vi "Nominal-Gate TimeOF.vi"(7 "Item ID":string) -> (1 "Error":bool, 2 "Gate Time":string, 3 "Nominal Frequency":string)   [LabVIEW 2023]
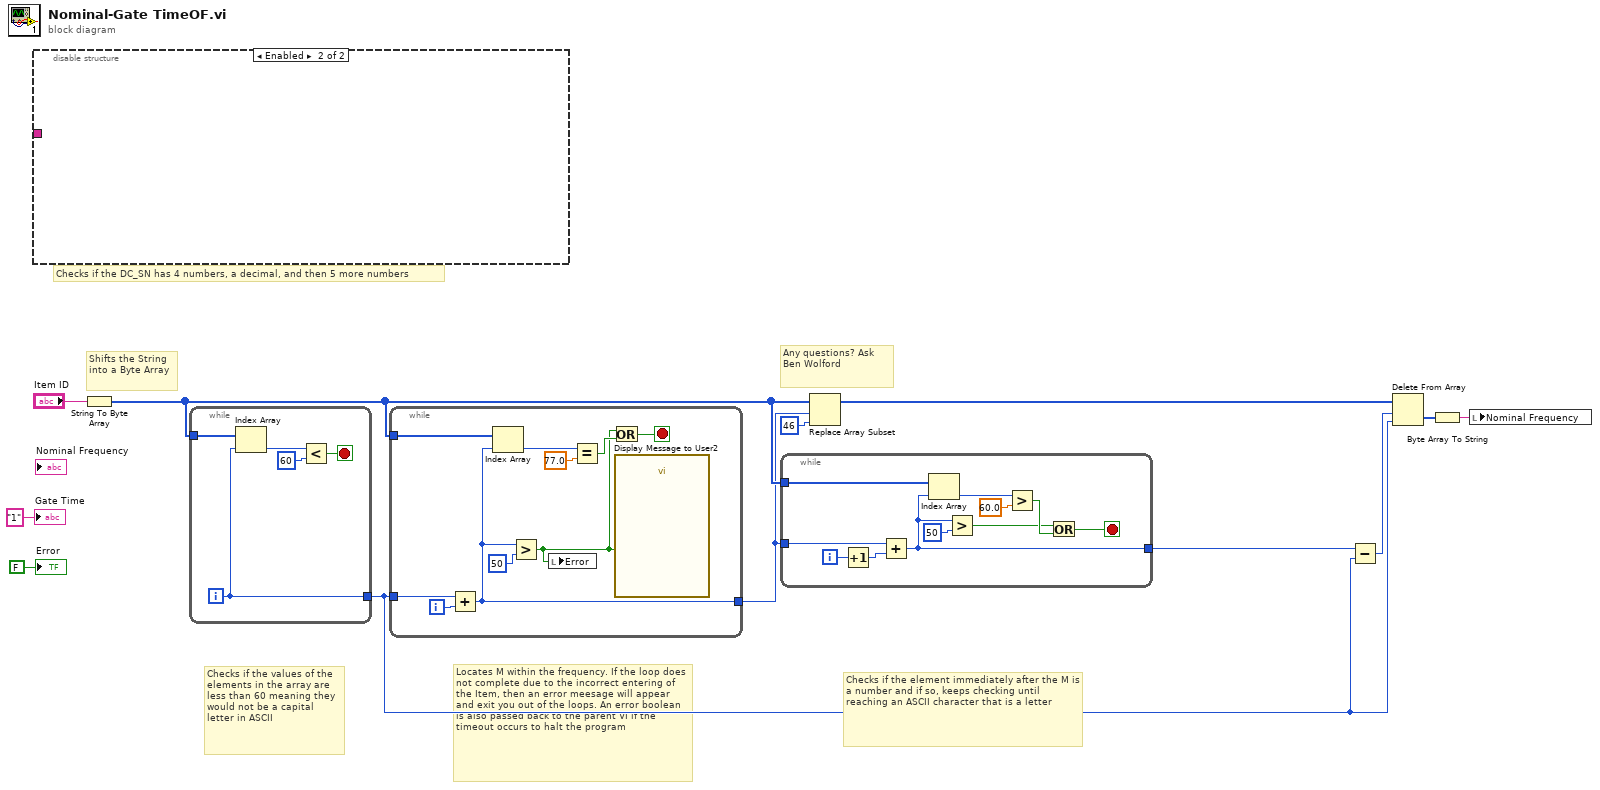
[diagram p0: block diagram]
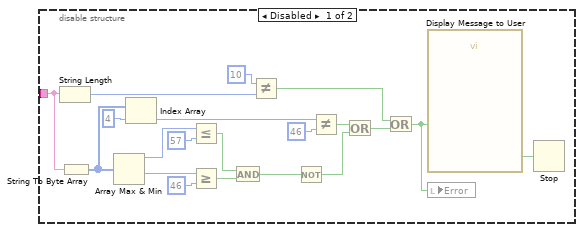
[diagram p2: hidden frame]
diagram:
  # "Checks if the element immediately after the M is a number and if so, keeps checking until reaching an ASCII character that is a letter"
  # "Locates M within the frequency. If the loop does not complete due to the incorrect entering of the Item, then an error meesage will appear and exit you out of the loops. An error boolean is also passed back to the parent VI if the timeout occurs to halt the program"
  # "Any questions? Ask Ben Wolford"
  # "Checks if the DC_SN has 4 numbers, a decimal, and then 5 more numbers"
  # "Checks if the values of the elements in the array are less than 60 meaning they would not be a capital letter in ASCII"
  # "Shifts the String into a Byte Array"
  n1 = disable-structure shown="Enabled" {
    disable-tunnel: _ -> [w13 _]
    frame Disabled {
      n2 = String Length(string=w13) -> (length=w19:i32)
      n3 = String To Byte Array(string=w13) -> (unsigned byte array=w26:u8[])
      n4 = Array Max & Min(array=w26) -> (max value=w28:u8, min value=w27:u8)  [unwired: 2 out]
      n5 = Index Array(array=w26, index=4) -> (element=w23:u8)
      n6 = Less Or Equal?(x=w28, y=u8 57) -> (x <= y?=w29:bool)
      n7 = Greater Or Equal?(x=w27, y=u8 46) -> (x >= y?=w30:bool)
      n8 = And(x=w29, y=w30) -> (x .and. y?=w31:bool)
      n9 = Not Equal?(x=10, y=w19) -> (x != y?=w20:bool)
      n10 = Not(x=w31) -> (.not. x?=w32:bool)
      n11 = Not Equal?(x=w23, y=u8 46) -> (x != y?=w25:bool)
      n12 = Or(x=w25, y=w32) -> (x .or. y?=w24:bool)
      n13 = Or(x=w20, y=w24) -> (x .or. y?=w21:bool)
      n14 = call "Display Message to User"("Enable"=w21) -> ("OK"=w22:bool)  [unwired: 9 in, 1 out]
      n15 = local write "Error"(w21) -> ()
      n16 = Stop(stop? (T)=w22) -> ()
    }
    frame Enabled {
    }
  }
  n17 = String To Byte Array(string="Item ID") -> (unsigned byte array=w10:u8[])
  n18 = while {
    tunnel: w10 -> [w37]
    tunnel: [w33] -> w1
    i -> [w33]
    stop <- w35 stop-if-true
    n19 = Index Array(array=w37, index=w33) -> (element=w36:u8)
    n20 = Less?(x=w36, y=u8 60) -> (x < y?=w35:bool)
  }
  n21 = while {
    tunnel: w10 -> [w45]
    tunnel: [w42] -> w6
    tunnel: w1 -> [w39]
    i -> [w38]
    stop <- w43 stop-if-true
    n22 = Add(x=w39, y=w38) -> (x+y=w42:i32)
    n23 = Index Array(array=w45, index=w42) -> (element=w46:u8)
    n24 = Greater?(x=w42, y=50) -> (0:w40:bool)
    n25 = local write "Error"(w40) -> ()
    n26 = Equal?(x=w46, y=77.0) -> (x = y?=w44:bool)
    n27 = Or(x=w40, y=w44) -> (x .or. y?=w43:bool)
    n28 = call "Display Message to User2"("Enable"=w40) -> ()  [unwired: 9 in, 2 out]
  }
  n29 = while {
    tunnel: w10 -> [w56]
    tunnel: [w49] -> w5
    tunnel: w6 -> [w55]
    i -> [w54]
    stop <- w51 stop-if-true
    n30 = Increment(x=w54) -> (x+1=w53:i32)
    n31 = Add(x=w55, y=w53) -> (x+y=w49:i32)
    n32 = Index Array(array=w56, index=w49) -> (element=w57:u8)
    n33 = Greater?(x=w49, y=50) -> (0:w48:bool)
    n34 = Greater?(x=w57, y=60.0) -> (0:w52:bool)
    n35 = Or(x=w48, y=w52) -> (x .or. y?=w51:bool)
  }
  n36 = Replace Array Subset(array=w10, new element=u8 46 ("new element/subarray"), index=w6) -> (w7:u8[])
  n37 = Subtract(x=w5, y=w1) -> (x-y=w4:i32)
  n38 = Delete From Array(array=w7, length=w4, index=w1) -> (deleted portion=w8:u8[])  [unwired: 1 out]
  n39 = Byte Array To String(unsigned byte array=w8) -> (string=w3:string)
  n40 = local write "Nominal Frequency"(w3) -> ()
  "Gate Time" <- "1" ("Gate Time")
  "Error" <- FALSE ("Error")
